vi "AssertControlValueEqual.vi"(0 "VI Reference In":refnum<vi>, 1 "Label":string, 5 "Control Name":string, 7 "Control Value":variant, 9 "Timeout(5 sec)":dbl=5.0, 11 "error out":errorcluster) -> (4 "VI Reference Out":refnum<vi>, 15 "error out":errorcluster)   [LabVIEW 2016]
doc: "<b>This VI asserts the value of controls in other VI.<b> \n\nThe input control name is given as a string , incase of path, use delimiters inbetween the path.\nThis VI gets the value of the control, untill the value is equal to the input value."
uses:
  AssertControlValueByPathString.vi
  <vilib>/addons/_JKI Toolkits/Caraya/classes/Assert/Assert Equal Value and Type_Variant.vi
  <vilib>/addons/_JKI Toolkits/Caraya/classes/Assert/Assert.lvclass
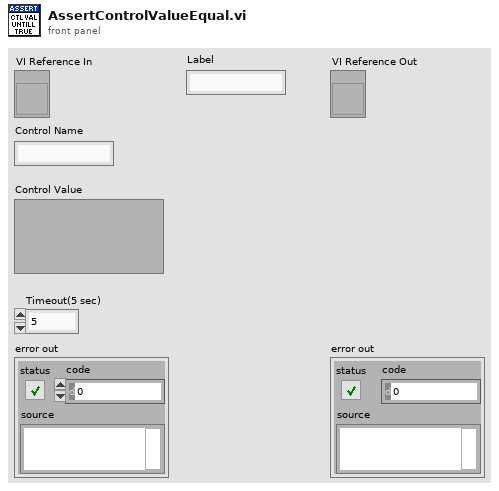
[diagram p1: front panel]
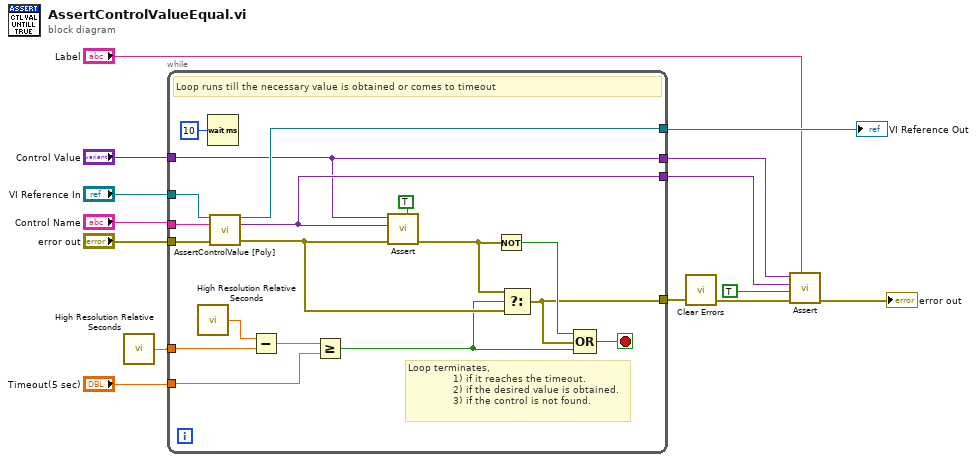
[diagram p0: block diagram]
diagram:
  n1 = call <vilib>:"High Resolution Relative Seconds.vi"() -> ("relative seconds"=w11:dbl)
  n2 = while {
    tunnel: "Control Name" -> [w31]
    tunnel: "VI Reference In" -> [w30]
    tunnel: "Control Value" -> [w19]
    tunnel: "Timeout(5 sec)" -> [w24]
    tunnel: [w27] -> w8
    tunnel: w11 -> [w29]
    tunnel: "error out" -> [w32]
    tunnel: [w16] -> w1
    tunnel: [w19] -> w6
    tunnel: [w20] -> w5
    stop <- w22 stop-if-true
    # "Loop terminates,\n               1) if it reaches the timeout.\n               2) if the desired value is obtained.\n               3) if the control is not found."
    # "Loop runs till the necessary value is obtained or comes to timeout"
    n3 = call <vilib>:"High Resolution Relative Seconds.vi"() -> ("relative seconds"=w28:dbl)
    n4 = Wait (ms)(milliseconds to wait=u32 10) -> ()  [unwired: 1 out]
    n5 = call-poly "AssertControlValue [Poly].vi"("VI Reference In"=w30, "Control Name"=w31, "error in"=w32) -> ("VI Reference Out"=w27:refnum<vi>, "Value"=w20:variant, "error out"=w23:errorcluster)  [unwired: 10 in]
    n6 = Subtract(x=w28, y=w29) -> (x-y=w25:dbl)
    n7 = Greater Or Equal?(x=w25, y=w24) -> (x >= y?=w18:bool)
    n8 = call-poly <vilib>:"Assert.vi"("Assert Only? (F)"=TRUE, "error in (no error)"=w23, "Y"=w20, "X"=w19) -> ("error out"=w21:errorcluster)  [unwired: 7 in]
    n9 = Not(x=w21) -> (.not. x?=w17:bool)
    n10 = Select(t=w21, s=w18, f=w23) -> (s? t:f=w16:errorcluster)
    n11 = Compound Arithmetic op=OR(w17, w16, w18) -> (w22:bool)
  }
  "VI Reference Out" <- w8
  n12 = call <vilib>:"Clear Errors.vi"("error in (no error)"=w1) -> ("error out"=w7:errorcluster)  [unwired: 5 in, 1 out]
  n13 = call-poly <vilib>:"Assert.vi"("Label"="Label", "error in (no error)"=w7, "Register with caller test (F)"=TRUE, "Y"=w5, "X"=w6) -> ("error out"=→"error out":errorcluster)  [unwired: 6 in]
